vi "Create Private Key.vi"(8 "error in (no error)":errorcluster, 11 "Agent Fixture in":refnum<class "Agent Fixture.lvclass">) -> (0 "error out":errorcluster, 3 "Agent Fixture out":refnum<class "Agent Fixture.lvclass">)   [LabVIEW 2013, in "libssh2_integration_tests.lvlib" / "Agent Fixture.lvclass"]
uses:
  Agent Fixture.lvclass
  Agent Fixture.lvclass/Agent Fixture.ctl
  libssh2_integration_tests.lvlib
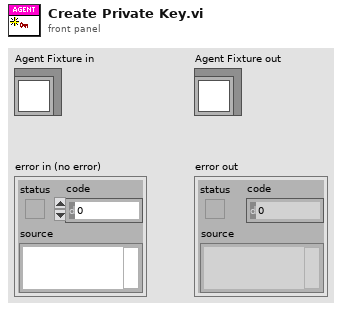
[diagram p1: front panel]
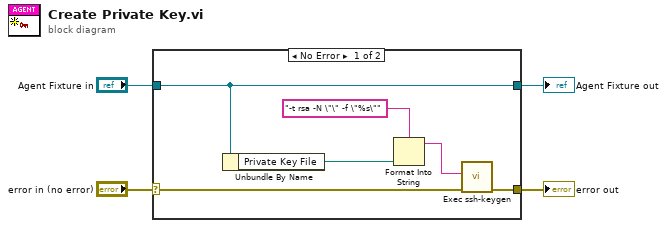
[diagram p0: block diagram]
diagram:
  n1 = case shown="No Error" "error in (no error)" {
    selector: "error in (no error)" -> [w8 w12]
    tunnel: [w6 w12] -> w3
    tunnel: [w7 w11] -> w1
    tunnel: "Agent Fixture in" -> [w7 w11]
    frame No Error {
      n2 = Unbundle By Name(w7) -> ("Private Key File"=w5:path)
      n3 = Format Into String(format string="-t rsa -N \"\" -f \"%s\"" ("arguments"), w5) -> (resulting string=w9:string)  [unwired: 2 in, 1 out]
      n4 = call "Exec ssh-keygen.vi"("error in (no error)"=w8, "arguments"=w9) -> ("error out"=w6:errorcluster)  [unwired: 9 in]
    }
    frame Error {
    }
  }
  "error out" <- w3
  "Agent Fixture out" <- w1
